vi "CTL_Level SpecRev3.vi"(6 "Index(n-1) In":i32[](array[numeric]), 7 "Full Cfg":T1, 8 "error in (no error)":errorcluster, 9 "Level IN inches":dbl=8.853199052567236, 11 "Drain!Fill":bool) -> (0 "error out":errorcluster, 2 "Enable":bool, 3 "Specs Out":T5, 4 "Index(n-1) Out":i32[](array[numeric]))   [LabVIEW 2024]
doc: "Determine the row index and Specification from the Config File Spec Table for the given level. \nAlso detemines the flag state for these Flags:\n Switch Zone = Resitor switch levels must occur in this zone\n R In Range Zone = Resistor value must be specified level\n R measure = When to take the measurement to record."
uses:
  Control Definitions/DEF_SpecsOut.ctl
  Control Definitions/Ded Spec RNG.ctl
  Control Definitions/Ded LUT_Status.ctl
  Control Definitions/Def PumpCtlRefs.ctl
  Control Definitions/Def_PumpSpeed.ctl
  Control Definitions/Def FullCfg.ctl
  Control Definitions/Def BenchCfg.ctl
  Control Definitions/Def Bench Status.ctl
  Control Definitions/Def TestState.ctl
panel:
  out "Index(n)":i32
  out "Boolean":bool=TRUE
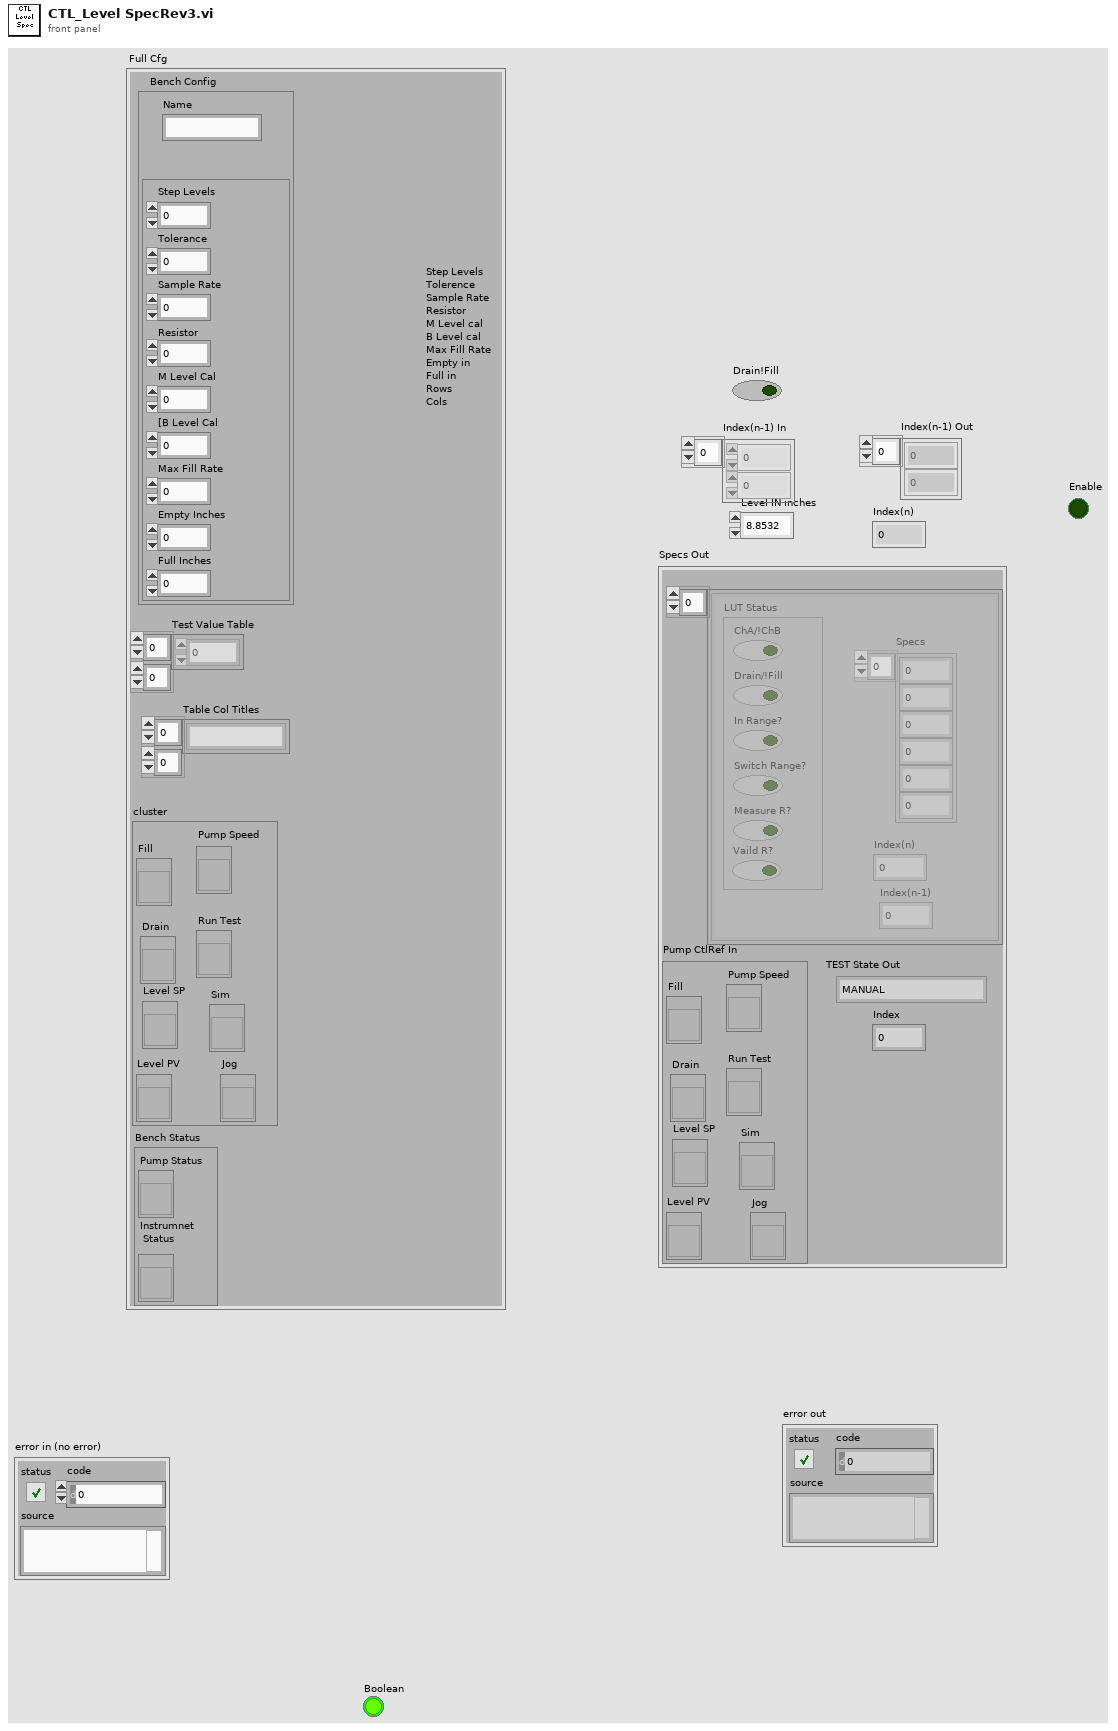
[diagram p1: front panel]
types:
  T1 = typedef "Def FullCfg.ctl" = cluster{"Bench Config":T2, "Test Value Table ":dbl[][], "Table Col Titles":string[][], "cluster":T3, "Bench Status":T4}
  T2 = typedef "Def BenchCfg.ctl" = cluster{"Name":string, cluster{"Step Levels":dbl, "Tolerance":dbl, "Sample Rate":dbl, "Resistor":dbl, "M Level Cal":dbl, "[B Level Cal":dbl, "Max Fill Rate":dbl, "Empty Inches":dbl, "Full Inches":dbl}}
  T3 = typedef "Def PumpCtlRefs.ctl" = cluster{"Fill ":refnum<vi>, "Drain":refnum<vi>, "Level PV":refnum<vi>, "Pump Speed":refnum<vi>, "Run Test":refnum<vi>, "Sim":refnum<vi>, "Jog":refnum<vi>, "Level SP":refnum<vi>}
  T4 = typedef "Def Bench Status.ctl" = cluster{"Pump Status":refnum<vi>, "Instrumnet\n Status":refnum<vi>}
  T5 = typedef "DEF_SpecsOut.ctl" = cluster{"aSpecsTable":T6[], "Pump CtlRef In":T3, "TEST State Out":T8, "Index":dbl}
  T6 = typedef "Ded Spec RNG.ctl" = cluster{"Specs":dbl[], "Index(n)":i32, "LUT Status":T7, "Index(n-1)":i32}
  T7 = typedef "Ded LUT_Status.ctl" = cluster{"ChA/!ChB":bool, "Drain/!Fill":bool, "In Range?":bool, "Switch Range?":bool, "Measure R?":bool, "Vaild R?":bool}
  T8 = typedef "Def TestState.ctl" = enum16{"MANUAL", "Start", "Pre-Fill", "Pre-Drain", "Init-Record", "Load Fill Spec", "Filling Hi", "Wait1", "Record Fill", "Load Drain Spec", "Draining Lo", "Wait2", "Record Drain", "Empty", "Done"}
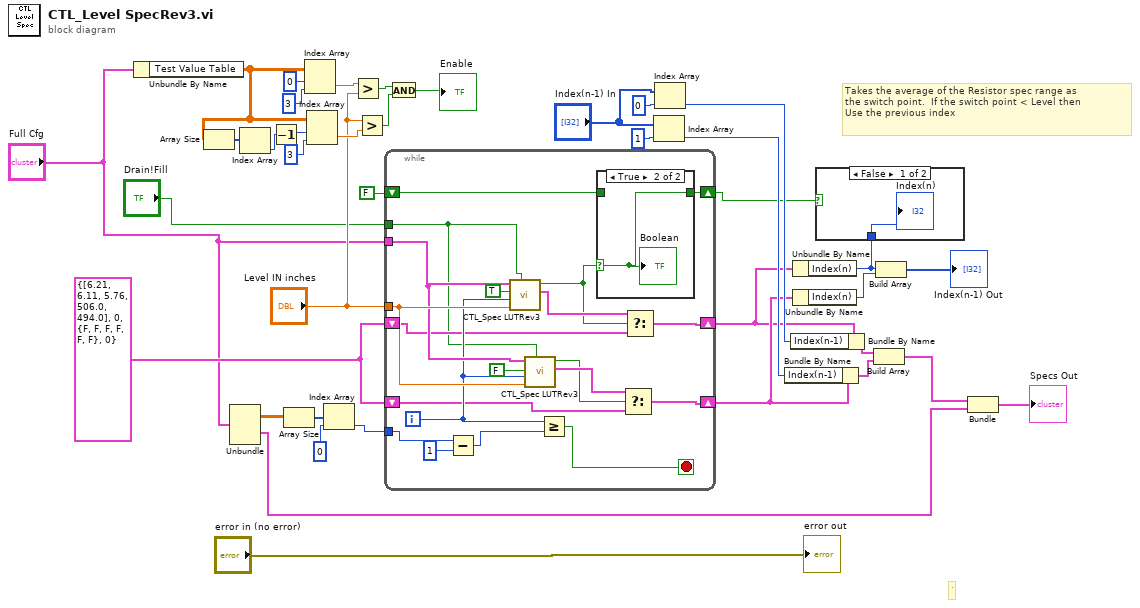
[diagram p0: block diagram]
diagram:
  w33 = T6 {"Specs"=[6.21, 6.11, 5.76, 506.0, 494.0], "Index(n)"=0, "LUT Status"={"ChA/!ChB"=FALSE, "Drain/!Fill"=FALSE, "In Range?"=FALSE, "Switch Range?"=FALSE, "Measure R?"=FALSE, "Vaild R?"=FALSE}, "Index(n-1)"=0} ("ChA Spec RNG")
  # "`"
  # "Takes the average of the Resistor spec range as \nthe switch point.  If the switch point < Level then \nUse the previous index"
  n1 = Unbundle By Name("Full Cfg") -> ("Test Value Table"=w9:dbl[][])
  n2 = Array Size(array=w9) -> (size(s)=w7:i32[])
  n3 = Unbundle("Full Cfg") -> ("Test Value Table"=w35:dbl[][], "cluster"=w4:T3)  [unwired: 3 out]
  n4 = Index Array(array=w7) -> (element=w6:i32)  [unwired: 1 in]
  n5 = Decrement(x=w6) -> (x-1=w8:i32)
  n6 = Array Size(array=w35) -> (size(s)=w38:i32[])
  n7 = Index Array(array=w9, index (row)=0, index (col)=3 ("disabled index (col)")) -> (element=w15:dbl)
  n8 = Index Array(array=w9, index (row)=w8, index (col)=3 ("disabled index (col)")) -> (element=w14:dbl)
  n9 = Index Array(array=w38, index=0) -> (element=w34:i32)
  n10 = Greater?(x=w15, y="Level IN inches") -> (0:w11:bool)
  n11 = Greater?(x="Level IN inches", y=w14) -> (0:w12:bool)
  n12 = while {
    tunnel: "Level IN inches" -> [w57]
    tunnel: "Full Cfg" -> [w55]
    tunnel: w34 -> [w42]
    shift-right: [w53] -> w24
    shift-left: w33 -> [w52]
    shift-right: [w48] -> w25
    shift-left: w33 -> [w47]
    shift-right: [w44] -> w19
    shift-left: FALSE -> [w43]
    tunnel: "Drain!Fill" -> [w39]
    i -> [w54]
    stop <- w51 stop-if-true
    n13 = Subtract(x=w42, y=1) -> (x-y=w40:i32)
    n14 = call "CTL_Spec LUTRev3.vi"("Drain!Fill"=w39, "Level IN inches"=w57, "Index"=w54, "ChA/!ChB"=TRUE, "Full Cfg"=w55) -> ("Spec RNG"=w46:T6, "In Range?"=w45:bool)  [unwired: 3 in, 2 out]
    n15 = call "CTL_Spec LUTRev3.vi"("Drain!Fill"=w39, "Level IN inches"=w57, "Index"=w54, "ChA/!ChB"=FALSE, "Full Cfg"=w55) -> ("Spec RNG"=w50:T6, "In Range?"=w49:bool)  [unwired: 3 in, 2 out]
    n16 = Greater Or Equal?(x=w54, y=w40) -> (x >= y?=w51:bool)
    n17 = case shown="True" w45 {
      selector: w45 -> [_ w60]
      tunnel: [w59 w60] -> w44
      tunnel: w43 -> [w59 _]
      frame False {
      }
      frame True {
        "Boolean" <- w60
      }
    }
    n18 = Select(t=w50, s=w49, f=w47) -> (s? t:f=w48:T6)
    n19 = Select(t=w46, s=w45, f=w52) -> (s? t:f=w53:T6)
  }
  n20 = And(x=w11, y=w12) -> (x .and. y?=→"Enable":bool)
  n21 = Index Array(array="Index(n-1) In", index=1) -> (element=w27:i32)
  n22 = Index Array(array="Index(n-1) In", index=0) -> (element=w26:i32)
  n23 = Bundle By Name(cluster=w25, "Index(n-1)"=w27) -> (w28:T6)
  n24 = Bundle By Name(cluster=w24, "Index(n-1)"=w26) -> (w29:T6)
  n25 = Unbundle By Name(w24) -> ("Index(n)"=w20:i32)
  n26 = Unbundle By Name(w25) -> ("Index(n)"=w23:i32)
  n27 = case shown="False" w19 {
    tunnel: w20 -> [w61 _]
    frame False {
      "Index(n)" <- w61
    }
    frame True {
    }
  }
  n28 = Build Array(w29, w28) -> (w5:T6[])
  n29 = Build Array(w20, w23) -> (→"Index(n-1) Out":i32[])
  n30 = Bundle(w5, "cluster"=w4) -> (→"Specs Out":cluster{T6[], "cluster":T3})  [unwired: 1 in]
  "error out" <- "error in (no error)"
